vi "Quaternion Average.vi"(8 "error in (no error)":errorcluster, 9 "Weights (Default: Empty = equal weights)":dbl[](array[numeric]), 11 "Quaternions":T1[](array[typedef])) -> (0 "error out":errorcluster, 3 "Average Quaternion":T1)   [LabVIEW 2020, in "ar.lvlib"]
doc: "Compute the Average of Quaternions with optional weights.\n\nSVD is used to compute an eigenvector which represents an weighted average of the input quaternions."
uses:
  ar.lvlib
  Quaternion.ctl
  common/common.lvlib
  common/bin/gartoolkit_ar_32-1.dll
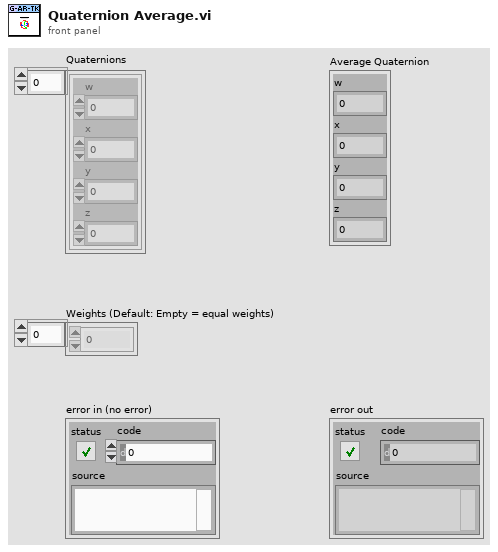
[diagram p1: front panel]
types:
  T1 = typedef "ar.lvlib/Quaternion.ctl" = cluster{"w":dbl, "x":dbl, "y":dbl, "z":dbl}
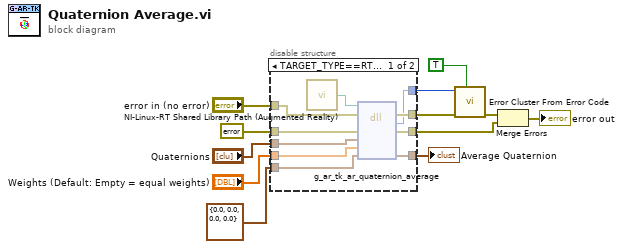
[diagram p0: block diagram]
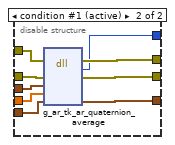
[diagram p2: hidden frame]
diagram:
  n1 = disable-structure shown="TARGET_TYPE==RT&&OS==Linux" {
    disable-tunnel: "error in (no error)" -> [w22 w31]
    disable-tunnel: errorcluster {"status"=FALSE, "code"=0, "source"=""} ("error constant") -> [w21 w30]
    disable-tunnel: "Quaternions" -> [w20 w29]
    disable-tunnel: "Weights (Default: Empty = equal weights)" -> [w19 w28]
    disable-tunnel: T1 {"w"=0.0, "x"=0.0, "y"=0.0, "z"=0.0} ("Quaternion") -> [w18 w27]
    disable-tunnel: [w17 w26] -> w5
    disable-tunnel: [w16 w25] -> w4
    disable-tunnel: [w15 w24] -> w3
    disable-tunnel: [w14 w23] -> w2
    frame condition #0 {
      n2 = call "NI-Linux-RT Shared Library Path (Augmented Reality).vi"() -> ("Path"=w13:path)
      n3 = dll-call lib="?" fn="g_ar_tk_ar_quaternion_average" ("g_ar_toolkit.*.*:g_ar_tk_image_copy")(path in=w13, error in=w22, "error_cluster"=w21, "input_quaternions"=w20, "Weights"=w19, "result_quaternion"=w18) -> (error out=w17:errorcluster, w16:i32, "error_cluster"=w15:errorcluster, "result_quaternion"=w14:T1)  [unwired: 3 in, 1 out]
    }
    frame condition #1 (active) {
      n4 = dll-call lib="C:/serenial/lib/g-augmented-reality-toolkit/LabVIEW/common/bin/gartoolkit_ar_*-1.*" fn="g_ar_tk_ar_quaternion_average" ("g_ar_toolkit.*.*:g_ar_tk_image_copy")(error in=w31, "error_cluster"=w30, "input_quaternions"=w29, "Weights"=w28, "result_quaternion"=w27) -> (error out=w26:errorcluster, w25:i32, "error_cluster"=w24:errorcluster, "result_quaternion"=w23:T1)  [unwired: 4 in, 1 out]
    }
  }
  "Average Quaternion" <- w2
  n5 = call <vilib>:"Error Cluster From Error Code.vi"("show call chain? (False)"=TRUE, "error in (no error)"=w5, "error code (0)"=w4) -> ("error out"=w12:errorcluster)  [unwired: 6 in]
  n6 = Merge Errors(w12, w3) -> (→"error out":errorcluster)
